vi "Affichage PokaenDex 1P.vi"() -> ()   [LabVIEW 2013]
uses:
  <vilib>/picture/picture.llb/Draw True-Color Pixmap.vi
panel:
  in  "Bouton OK 2":bool
  in  "Port USB en réception":refnum<visa-resource-name>="ASRL1::INSTR"
  out "Cache rouge":picture
  out "Image 2D":picture
  out "sign 1":u32
  out "Distance cible":string
  out "Cam D détect":bool
  out "2 cam détect":bool
  out "Cam G détect":bool
  in  "2D/3D":bool caption="Booléen 5"
  in  "Booléen":bool
  out "Ennemi":bool
  out "Ami":bool
  out "Cache gris":picture
  out "Nom du Pokaenmon":string
  out "Pokeanmon détécté !":bool
  in  "stop":bool
  out "Image Pokaenmon":picture
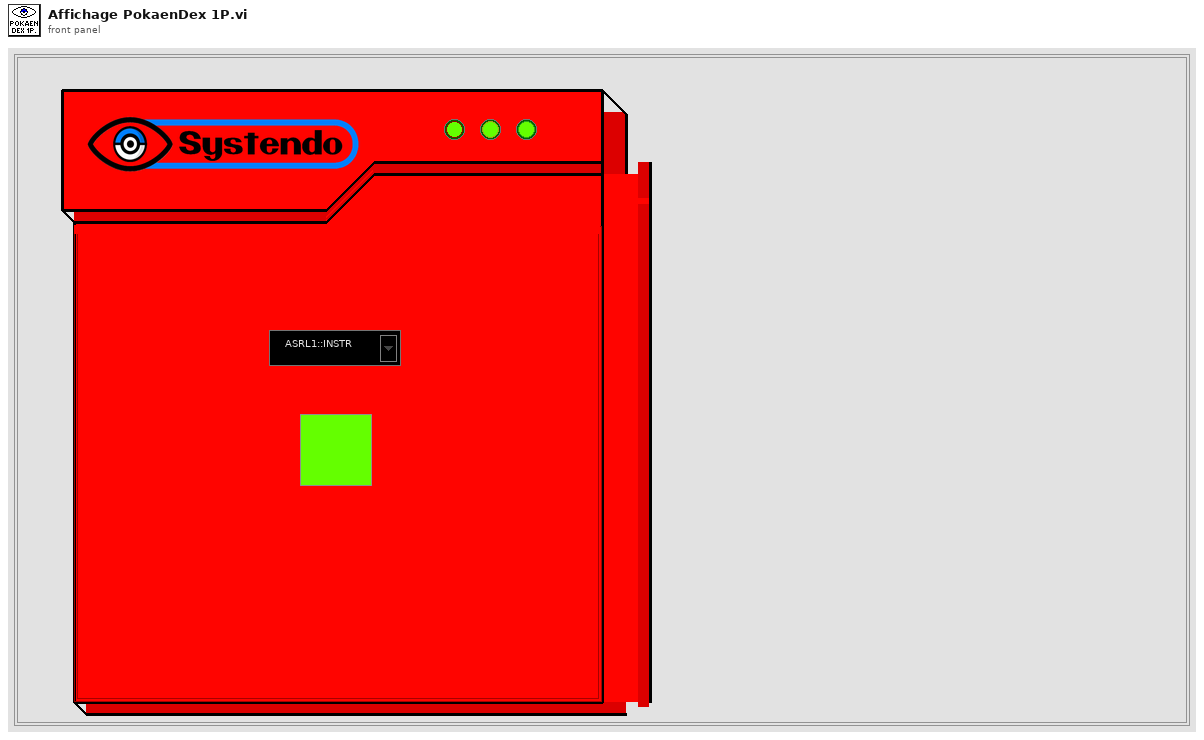
[diagram p1: front panel]
types:
  T1 = cluster{"left":i16, "top":i16, "right":i16, "bottom":i16}
  T2 = cluster{"Pokaenmon détecté":bool, "Signature":u32, "x":dbl, "y ":dbl, "Longueur":dbl, "Hauteur":dbl}
  T3 = cluster{"Données Caméra G":cluster{dbl, dbl, dbl, dbl}, "Données Caméra D":cluster{dbl, dbl, dbl, dbl}}
  T4 = typedef "imagedata.ctl" = cluster{"image type":i32, "image depth":i32, "image":u8[], "mask":u8[], "colors":u32[], "Rectangle":cluster{"left":i16, "top":i16, "right":i16, "bottom":i16}}
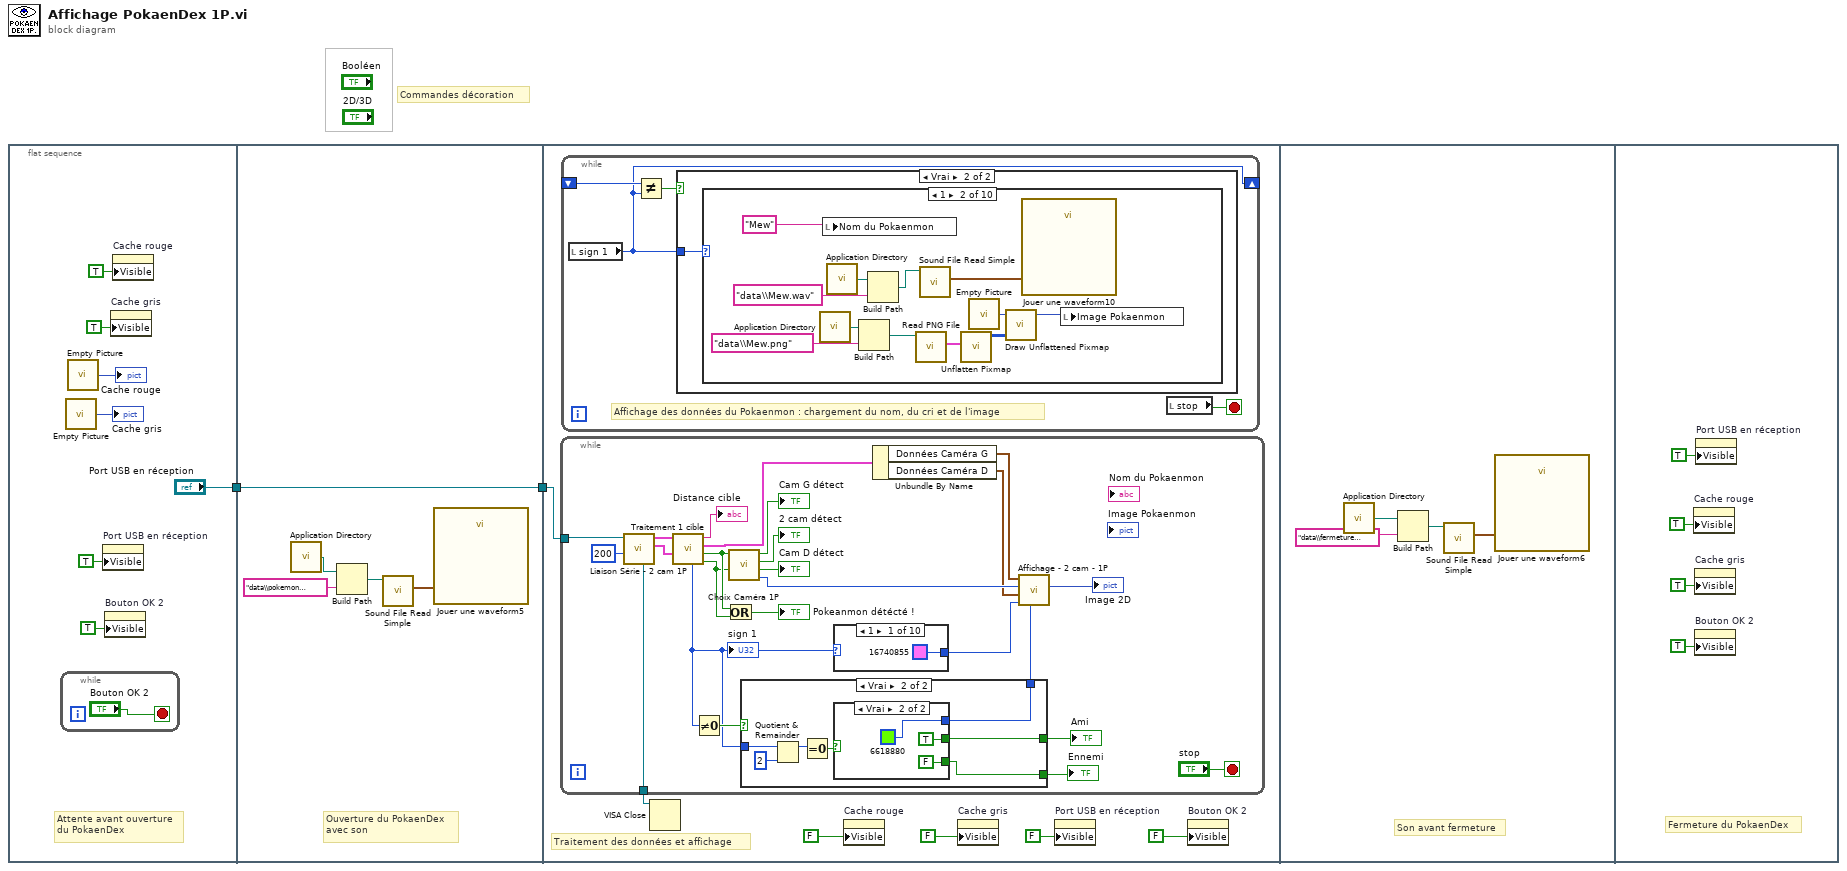
[diagram p0: block diagram]
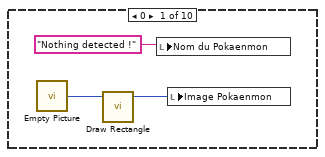
[diagram p3: hidden frame]
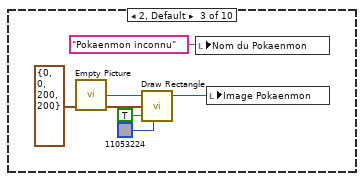
[diagram p4: hidden frame]
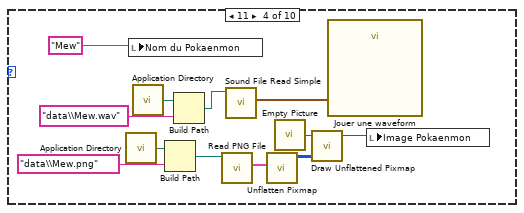
[diagram p5: hidden frame]
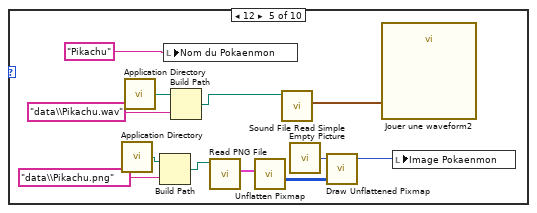
[diagram p6: hidden frame]
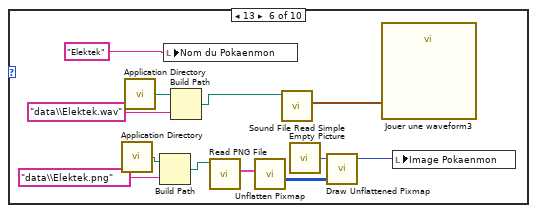
[diagram p7: hidden frame]
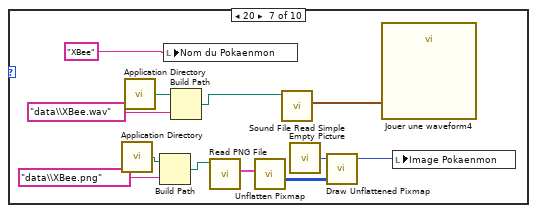
[diagram p8: hidden frame]
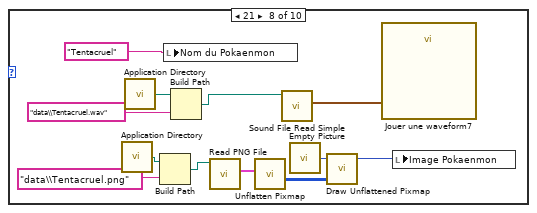
[diagram p9: hidden frame]
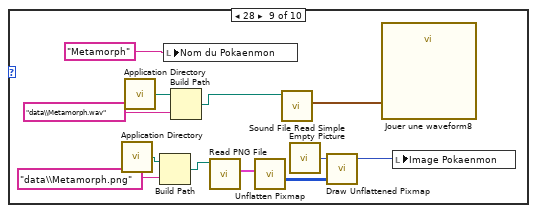
[diagram p10: hidden frame]
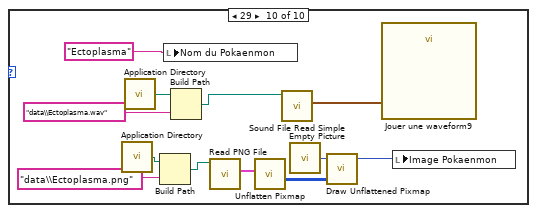
[diagram p11: hidden frame]
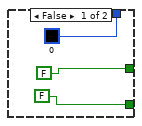
[diagram p12: hidden frame]
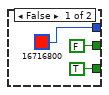
[diagram p13: hidden frame]
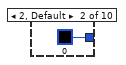
[diagram p14: hidden frame]
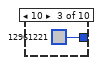
[diagram p15: hidden frame]
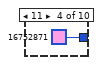
[diagram p16: hidden frame]
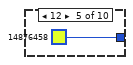
[diagram p17: hidden frame]
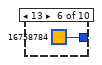
[diagram p18: hidden frame]
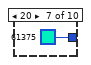
[diagram p19: hidden frame]
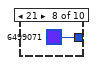
[diagram p20: hidden frame]
diagram:
  # "Commandes décoration"
  n1 = flat-sequence {
    tunnel: ["Port USB en réception"] -> w2
    tunnel: w2 -> [w15]
    tunnel: [w15] -> w1
    tunnel: w1 -> [w20]
    frame #0 {
      # "Attente avant ouverture\ndu PokaenDex"
      n2 = while {
        stop <- "Bouton OK 2" stop-if-true
      }
      n3 = call "Empty Picture"() -> ("empty picture"=→"Cache gris":picture)
      n4 = call "Empty Picture"() -> ("empty picture"=→"Cache rouge":picture)
      n5 = property on="Port USB en réception" class="NomVISA"("Visible"=TRUE) -> ()  [unwired: 2 in, 2 out]
      n6 = property on="Bouton OK 2" class="Bool"("Visible"=TRUE) -> ()  [unwired: 2 in, 2 out]
      n7 = property on="Cache gris" class="Image"("Visible"=TRUE) -> ()  [unwired: 2 in, 2 out]
      n8 = property on="Cache rouge" class="Image"("Visible"=TRUE) -> ()  [unwired: 2 in, 2 out]
    }
    frame #1 {
      # "Ouverture du PokaenDex\navec son"
      n9 = call <vilib>:"Application Directory.vi"() -> ("Application Directory"=w11:path)
      n10 = Build Path(base path=w11, name or relative path="data\\pokemon ouverture.wav") -> (appended path=w12:path)
      n11 = call <vilib>:"Sound File Read Simple.vi"("path"=w12) -> ("data"=w14:waveform(dbl)[])  [unwired: 7 in, 3 out]
      n12 = call "Jouer une waveform5"("Data"=w14) -> ()  [unwired: 18 in, 1 out]
    }
    frame #2 {
      # "Traitement des données et affichage"
      n13 = while {
        tunnel: w20 -> [w147]
        tunnel: [w146] -> w21
        stop <- "stop" stop-if-true
        n14 = call "Liaison Série - 2 cam 1P.vi"("timeout (ms)"=u32 200 ("timeout (10sec)"), "Port USB en réception"=w147) -> ("Indications pokaenmon D"=w139:T2, "Indications pokaenmon G"=w145:T2, "Nom VISA en sortie"=w146:refnum<visa-resource-name>)  [unwired: 7 in]
        n15 = call "Traitement 1 cible.vi"("Indications Pokaenmon D"=w139, "Indications Pokaenmon G"=w145) -> ("D détect"=w141:bool, "G détect"=w142:bool, "Données caméras"=w132:T3, "Distance"=→"Distance cible":string, "Signature"=w135:u32)  [unwired: 5 in]
        "sign 1" <- w135
        n16 = Not Equal To 0?(x=w135) -> (x != 0?=w136:bool)
        n17 = Or(x=w142, y=w141) -> (x .or. y?=→"Pokeanmon détécté !":bool)
        n18 = call "Choix Caméra 1P.vi"("Detecté caméra D"=w141, "Detecté caméra G"=w142) -> ("Choix"=w153:u16, "Detecté caméra D"=→"Cam D détect":bool, "Detecté caméra G et D"=→"2 cam détect":bool, "Detecté caméra G"=→"Cam G détect":bool)  [unwired: 6 in]
        n19 = case shown="Vrai" w136 {
          tunnel: w135 -> [_ w162]
          tunnel: [u32 0 ("Couleur rectangle") w161] -> w137
          tunnel: [FALSE w160] -> w134
          tunnel: [FALSE w159] -> w133
          frame False {
          }
          frame True {
            n20 = Quotient & Remainder(x=w162, y=2) -> (x-y*floor(x/y)=w164:u32)  [unwired: 1 out]
            n21 = Equal To 0?(x=w164) -> (x = 0?=w165:bool)
            n22 = case shown="Vrai" w165 {
              tunnel: [FALSE TRUE] -> w160
              tunnel: [TRUE FALSE] -> w159
              tunnel: [u32 16716800 ("Couleur rectangle") u32 6618880 ("Couleur rectangle")] -> w161
              frame False {
              }
              frame True {
              }
            }
          }
        }
        "Ami" <- w134
        "Ennemi" <- w133
        n23 = case shown="1" w135 {
          tunnel: [u32 16740855 ("Couleur rectangle") u32 0 ("Couleur rectangle") u32 12961221 ("Couleur rectangle") u32 16752871 ("Couleur rectangle") u32 14876458 ("Couleur rectangle") u32 16758784 ("Couleur rectangle") u32 61375 ("Couleur rectangle") u32 6499071 ("Couleur rectangle") u32 15663254 ("Couleur rectangle") u32 10092783 ("Couleur rectangle")] -> w154
          frame 1 {
          }
          frame 2, Default {
          }
          frame 10 {
          }
          frame 11 {
          }
          frame 12 {
          }
          frame 13 {
          }
          frame 20 {
          }
          frame 21 {
          }
          frame 29 {
          }
          frame 28 {
          }
        }
        n24 = Unbundle By Name(w132) -> ("Données Caméra G"=w143:cluster{dbl, dbl, dbl, dbl}, "Données Caméra D"=w144:cluster{dbl, dbl, dbl, dbl})
        n25 = call "Affichage - 2 cam - 1P.vi"("Couleur fond"=w137, "Couleur rectangle"=w154, "Caméra D"=w144, "Choix cam"=w153, "Caméra G"=w143) -> ("Image 2D"=→"Image 2D":picture)  [unwired: 6 in]
      }
      n26 = while {
        shift-right: [w22] -> _
        shift-left: _ -> [w24]
        stop <- w25 stop-if-true
        # "Affichage des données du Pokaenmon : chargement du nom, du cri et de l'image"
        n27 = local read "sign 1"() -> (w22:u32)
        n28 = Not Equal?(x=w24, y=w22) -> (x != y?=w23:bool)
        n29 = case shown="Vrai" w23 {
          tunnel: w22 -> [_ w26]
          frame False {
          }
          frame True {
            n30 = case shown="1" w26 {
              frame 0 {
                n31 = call "Empty Picture"() -> ("empty picture"=w29:picture)
                n32 = call <vilib>:"Draw Rectangle.vi"("picture"=w29) -> ("new picture"=w27:picture)  [unwired: 8 in]
                n33 = local write "Nom du Pokaenmon"("Nothing detected !") -> ()
                n34 = local write "Image Pokaenmon"(w27) -> ()
              }
              frame 1 {
                n35 = call <vilib>:"Application Directory.vi"() -> ("Application Directory"=w30:path)
                n36 = local write "Nom du Pokaenmon"("Mew") -> ()
                n37 = call <vilib>:"Application Directory.vi"() -> ("Application Directory"=w31:path)
                n38 = Build Path(base path=w30, name or relative path="data\\Mew.png") -> (appended path=w32:path)
                n39 = Build Path(base path=w31, name or relative path="data\\Mew.wav") -> (appended path=w34:path)
                n40 = call <vilib>:"Read PNG File.vi"("path to PNG file"=w32) -> ("image data"=w40:T4)  [unwired: 8 in, 2 out]
                n41 = call <vilib>:"Sound File Read Simple.vi"("path"=w34) -> ("data"=w36:waveform(dbl)[])  [unwired: 7 in, 3 out]
                n42 = call <vilib>:"Unflatten Pixmap.vi"("image data"=w40) -> ("24-bit pixmap"=w39:u32[][])  [unwired: 4 in, 6 out]
                n43 = call "Empty Picture"() -> ("empty picture"=w41:picture)
                n44 = call-poly <vilib>:"Draw Unflattened Pixmap.vi"("picture"=w41, "data (RGB format)"=w39) -> ("new picture"=w37:picture)  [unwired: 7 in]
                n45 = call "Jouer une waveform10"("Data"=w36) -> ()  [unwired: 18 in, 1 out]
                n46 = local write "Image Pokaenmon"(w37) -> ()
              }
              frame 2, Default {
                n47 = call "Empty Picture"() -> ("empty picture"=w47:picture)
                n48 = call <vilib>:"Draw Rectangle.vi"("picture"=w47, "rect"=T1 {"left"=0, "top"=0, "right"=200, "bottom"=200}, "fill?(F)"=TRUE, "color(black)"=u32 11053224) -> ("new picture"=w45:picture)  [unwired: 5 in]
                n49 = local write "Nom du Pokaenmon"("Pokaenmon inconnu") -> ()
                n50 = local write "Image Pokaenmon"(w45) -> ()
              }
              frame 11 {
                n51 = call <vilib>:"Application Directory.vi"() -> ("Application Directory"=w48:path)
                n52 = local write "Nom du Pokaenmon"("Mew") -> ()
                n53 = call <vilib>:"Application Directory.vi"() -> ("Application Directory"=w49:path)
                n54 = Build Path(base path=w48, name or relative path="data\\Mew.png") -> (appended path=w50:path)
                n55 = Build Path(base path=w49, name or relative path="data\\Mew.wav") -> (appended path=w52:path)
                n56 = call <vilib>:"Read PNG File.vi"("path to PNG file"=w50) -> ("image data"=w58:T4)  [unwired: 8 in, 2 out]
                n57 = call <vilib>:"Sound File Read Simple.vi"("path"=w52) -> ("data"=w54:waveform(dbl)[])  [unwired: 7 in, 3 out]
                n58 = call <vilib>:"Unflatten Pixmap.vi"("image data"=w58) -> ("24-bit pixmap"=w57:u32[][])  [unwired: 4 in, 6 out]
                n59 = call "Empty Picture"() -> ("empty picture"=w59:picture)
                n60 = call-poly <vilib>:"Draw Unflattened Pixmap.vi"("picture"=w59, "data (RGB format)"=w57) -> ("new picture"=w55:picture)  [unwired: 7 in]
                n61 = call "Jouer une waveform"("Data"=w54) -> ()  [unwired: 18 in, 1 out]
                n62 = local write "Image Pokaenmon"(w55) -> ()
              }
              frame 12 {
                n63 = call <vilib>:"Application Directory.vi"() -> ("Application Directory"=w60:path)
                n64 = call <vilib>:"Application Directory.vi"() -> ("Application Directory"=w61:path)
                n65 = Build Path(base path=w60, name or relative path="data\\Pikachu.png") -> (appended path=w64:path)
                n66 = local write "Nom du Pokaenmon"("Pikachu") -> ()
                n67 = Build Path(base path=w61, name or relative path="data\\Pikachu.wav") -> (appended path=w62:path)
                n68 = call <vilib>:"Read PNG File.vi"("path to PNG file"=w64) -> ("image data"=w70:T4)  [unwired: 8 in, 2 out]
                n69 = call <vilib>:"Unflatten Pixmap.vi"("image data"=w70) -> ("24-bit pixmap"=w69:u32[][])  [unwired: 4 in, 6 out]
                n70 = call <vilib>:"Sound File Read Simple.vi"("path"=w62) -> ("data"=w66:waveform(dbl)[])  [unwired: 7 in, 3 out]
                n71 = call "Empty Picture"() -> ("empty picture"=w71:picture)
                n72 = call-poly <vilib>:"Draw Unflattened Pixmap.vi"("picture"=w71, "data (RGB format)"=w69) -> ("new picture"=w67:picture)  [unwired: 7 in]
                n73 = call "Jouer une waveform2"("Data"=w66) -> ()  [unwired: 18 in, 1 out]
                n74 = local write "Image Pokaenmon"(w67) -> ()
              }
              frame 13 {
                n75 = call <vilib>:"Application Directory.vi"() -> ("Application Directory"=w72:path)
                n76 = call <vilib>:"Application Directory.vi"() -> ("Application Directory"=w73:path)
                n77 = Build Path(base path=w72, name or relative path="data\\Elektek.png") -> (appended path=w76:path)
                n78 = local write "Nom du Pokaenmon"("Elektek") -> ()
                n79 = Build Path(base path=w73, name or relative path="data\\Elektek.wav") -> (appended path=w74:path)
                n80 = call <vilib>:"Read PNG File.vi"("path to PNG file"=w76) -> ("image data"=w82:T4)  [unwired: 8 in, 2 out]
                n81 = call <vilib>:"Unflatten Pixmap.vi"("image data"=w82) -> ("24-bit pixmap"=w81:u32[][])  [unwired: 4 in, 6 out]
                n82 = call <vilib>:"Sound File Read Simple.vi"("path"=w74) -> ("data"=w78:waveform(dbl)[])  [unwired: 7 in, 3 out]
                n83 = call "Empty Picture"() -> ("empty picture"=w83:picture)
                n84 = call-poly <vilib>:"Draw Unflattened Pixmap.vi"("picture"=w83, "data (RGB format)"=w81) -> ("new picture"=w79:picture)  [unwired: 7 in]
                n85 = call "Jouer une waveform3"("Data"=w78) -> ()  [unwired: 18 in, 1 out]
                n86 = local write "Image Pokaenmon"(w79) -> ()
              }
              frame 20 {
                n87 = call <vilib>:"Application Directory.vi"() -> ("Application Directory"=w84:path)
                n88 = call <vilib>:"Application Directory.vi"() -> ("Application Directory"=w85:path)
                n89 = Build Path(base path=w84, name or relative path="data\\XBee.png") -> (appended path=w88:path)
                n90 = local write "Nom du Pokaenmon"("XBee") -> ()
                n91 = Build Path(base path=w85, name or relative path="data\\XBee.wav") -> (appended path=w86:path)
                n92 = call <vilib>:"Read PNG File.vi"("path to PNG file"=w88) -> ("image data"=w94:T4)  [unwired: 8 in, 2 out]
                n93 = call <vilib>:"Unflatten Pixmap.vi"("image data"=w94) -> ("24-bit pixmap"=w93:u32[][])  [unwired: 4 in, 6 out]
                n94 = call <vilib>:"Sound File Read Simple.vi"("path"=w86) -> ("data"=w90:waveform(dbl)[])  [unwired: 7 in, 3 out]
                n95 = call "Empty Picture"() -> ("empty picture"=w95:picture)
                n96 = call-poly <vilib>:"Draw Unflattened Pixmap.vi"("picture"=w95, "data (RGB format)"=w93) -> ("new picture"=w91:picture)  [unwired: 7 in]
                n97 = call "Jouer une waveform4"("Data"=w90) -> ()  [unwired: 18 in, 1 out]
                n98 = local write "Image Pokaenmon"(w91) -> ()
              }
              frame 21 {
                n99 = call <vilib>:"Application Directory.vi"() -> ("Application Directory"=w96:path)
                n100 = call <vilib>:"Application Directory.vi"() -> ("Application Directory"=w97:path)
                n101 = Build Path(base path=w96, name or relative path="data\\Tentacruel.png") -> (appended path=w100:path)
                n102 = local write "Nom du Pokaenmon"("Tentacruel") -> ()
                n103 = Build Path(base path=w97, name or relative path="data\\Tentacruel.wav") -> (appended path=w98:path)
                n104 = call <vilib>:"Read PNG File.vi"("path to PNG file"=w100) -> ("image data"=w106:T4)  [unwired: 8 in, 2 out]
                n105 = call <vilib>:"Unflatten Pixmap.vi"("image data"=w106) -> ("24-bit pixmap"=w105:u32[][])  [unwired: 4 in, 6 out]
                n106 = call <vilib>:"Sound File Read Simple.vi"("path"=w98) -> ("data"=w102:waveform(dbl)[])  [unwired: 7 in, 3 out]
                n107 = call "Empty Picture"() -> ("empty picture"=w107:picture)
                n108 = call-poly <vilib>:"Draw Unflattened Pixmap.vi"("picture"=w107, "data (RGB format)"=w105) -> ("new picture"=w103:picture)  [unwired: 7 in]
                n109 = call "Jouer une waveform7"("Data"=w102) -> ()  [unwired: 18 in, 1 out]
                n110 = local write "Image Pokaenmon"(w103) -> ()
              }
              frame 28 {
                n111 = call <vilib>:"Application Directory.vi"() -> ("Application Directory"=w108:path)
                n112 = call <vilib>:"Application Directory.vi"() -> ("Application Directory"=w109:path)
                n113 = Build Path(base path=w108, name or relative path="data\\Metamorph.png") -> (appended path=w112:path)
                n114 = local write "Nom du Pokaenmon"("Metamorph") -> ()
                n115 = Build Path(base path=w109, name or relative path="data\\Metamorph.wav") -> (appended path=w110:path)
                n116 = call <vilib>:"Read PNG File.vi"("path to PNG file"=w112) -> ("image data"=w118:T4)  [unwired: 8 in, 2 out]
                n117 = call <vilib>:"Unflatten Pixmap.vi"("image data"=w118) -> ("24-bit pixmap"=w117:u32[][])  [unwired: 4 in, 6 out]
                n118 = call <vilib>:"Sound File Read Simple.vi"("path"=w110) -> ("data"=w114:waveform(dbl)[])  [unwired: 7 in, 3 out]
                n119 = call "Empty Picture"() -> ("empty picture"=w119:picture)
                n120 = call-poly <vilib>:"Draw Unflattened Pixmap.vi"("picture"=w119, "data (RGB format)"=w117) -> ("new picture"=w115:picture)  [unwired: 7 in]
                n121 = call "Jouer une waveform8"("Data"=w114) -> ()  [unwired: 18 in, 1 out]
                n122 = local write "Image Pokaenmon"(w115) -> ()
              }
              frame 29 {
                n123 = call <vilib>:"Application Directory.vi"() -> ("Application Directory"=w120:path)
                n124 = call <vilib>:"Application Directory.vi"() -> ("Application Directory"=w121:path)
                n125 = Build Path(base path=w120, name or relative path="data\\Ectoplasma.png") -> (appended path=w124:path)
                n126 = local write "Nom du Pokaenmon"("Ectoplasma") -> ()
                n127 = Build Path(base path=w121, name or relative path="data\\Ectoplasma.wav") -> (appended path=w122:path)
                n128 = call <vilib>:"Read PNG File.vi"("path to PNG file"=w124) -> ("image data"=w130:T4)  [unwired: 8 in, 2 out]
                n129 = call <vilib>:"Unflatten Pixmap.vi"("image data"=w130) -> ("24-bit pixmap"=w129:u32[][])  [unwired: 4 in, 6 out]
                n130 = call <vilib>:"Sound File Read Simple.vi"("path"=w122) -> ("data"=w126:waveform(dbl)[])  [unwired: 7 in, 3 out]
                n131 = call "Empty Picture"() -> ("empty picture"=w131:picture)
                n132 = call-poly <vilib>:"Draw Unflattened Pixmap.vi"("picture"=w131, "data (RGB format)"=w129) -> ("new picture"=w127:picture)  [unwired: 7 in]
                n133 = call "Jouer une waveform9"("Data"=w126) -> ()  [unwired: 18 in, 1 out]
                n134 = local write "Image Pokaenmon"(w127) -> ()
              }
            }
          }
        }
        n135 = local read "stop"() -> (w25:bool)
      }
      n136 = VISA Close(VISA resource name=w21) -> ()  [unwired: 1 in, 1 out]
      n137 = property on="Cache rouge" class="Image"("Visible"=FALSE) -> ()  [unwired: 2 in, 2 out]
      n138 = property on="Cache gris" class="Image"("Visible"=FALSE) -> ()  [unwired: 2 in, 2 out]
      n139 = property on="Port USB en réception" class="NomVISA"("Visible"=FALSE) -> ()  [unwired: 2 in, 2 out]
      n140 = property on="Bouton OK 2" class="Bool"("Visible"=FALSE) -> ()  [unwired: 2 in, 2 out]
    }
    frame #3 {
      # "Son avant fermeture"
      n141 = call <vilib>:"Application Directory.vi"() -> ("Application Directory"=w182:path)
      n142 = Build Path(base path=w182, name or relative path="data\\fermeture pokedex.wav") -> (appended path=w183:path)
      n143 = call <vilib>:"Sound File Read Simple.vi"("path"=w183) -> ("data"=w185:waveform(dbl)[])  [unwired: 7 in, 3 out]
      n144 = call "Jouer une waveform6"("Data"=w185) -> ()  [unwired: 18 in, 1 out]
    }
    frame #4 {
      # "Fermeture du PokaenDex"
      n145 = property on="Cache rouge" class="Image"("Visible"=TRUE) -> ()  [unwired: 2 in, 2 out]
      n146 = property on="Cache gris" class="Image"("Visible"=TRUE) -> ()  [unwired: 2 in, 2 out]
      n147 = property on="Bouton OK 2" class="Bool"("Visible"=TRUE) -> ()  [unwired: 2 in, 2 out]
      n148 = property on="Port USB en réception" class="NomVISA"("Visible"=TRUE) -> ()  [unwired: 2 in, 2 out]
    }
  }
